vi "FindMovingObjects_Xiang.vi"(6 "Initialize?":bool, 7 "Settings":T2={"Objects"=0, "Threshold"=128, "Reject Border"=FALSE, "Fill Holes"=FALSE, "Min Object Size"=FALSE, "Min Size"=3, "Max Object Size"=FALSE, "Max Size"=100, "Show Search Area"=FALSE, "Show Center"=TRUE, "Show Bounding Box"=TRUE} {"Objects" items=["Bright Objects", "Dark Objects"]; "Threshold" min=1 max=999999999 step=1; "Max Size" min=1 max=999999999 step=1; "Min Size" min=1 max=999999999 step=1}, 8 "Buffer Length":i32=50, 10 "Image Dst":T3, 11 "Image Src":T3) -> (2 "Objects":T1(array[cluster]) {"Aspect Ratio" format="%.2f"; "Orientation" format="%.2f"; "Area" format="%.2f"; "Object Center"."Y" format="%.2f"; "Object Center"."X" format="%.2f"}, 3 "Image Dst Out":T3)   [LabVIEW 2017]
uses:
  <vilib>/vision/Image Controls.llb/IMAQ Image.ctl
  <vilib>/vision/NI_Vision_Development_Module.lvlib
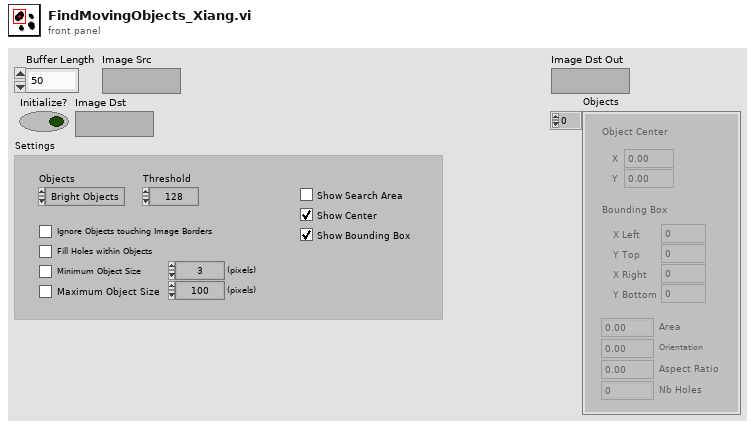
[diagram p1: front panel]
types:
  T1 = cluster{"Object Center":cluster{"X":sgl, "Y":sgl}, "Bounding Box":cluster{"X Left":i32, "Y Top":i32, "X Right":i32, "Y Bottom":i32}, "Area":sgl, "Orientation":sgl, "Aspect Ratio":sgl, "Nb Holes":i32}[]
  T2 = cluster{"Objects":u16, "Threshold":i32, "Reject Border":bool, "Fill Holes":bool, "Min Object Size":bool, "Min Size":i32, "Max Object Size":bool, "Max Size":i32, "Show Search Area":bool, "Show Center":bool, "Show Bounding Box":bool}
  T3 = typedef "IMAQ Image.ctl" = refnum<image>
  T4 = typedef "Image Type" = u32
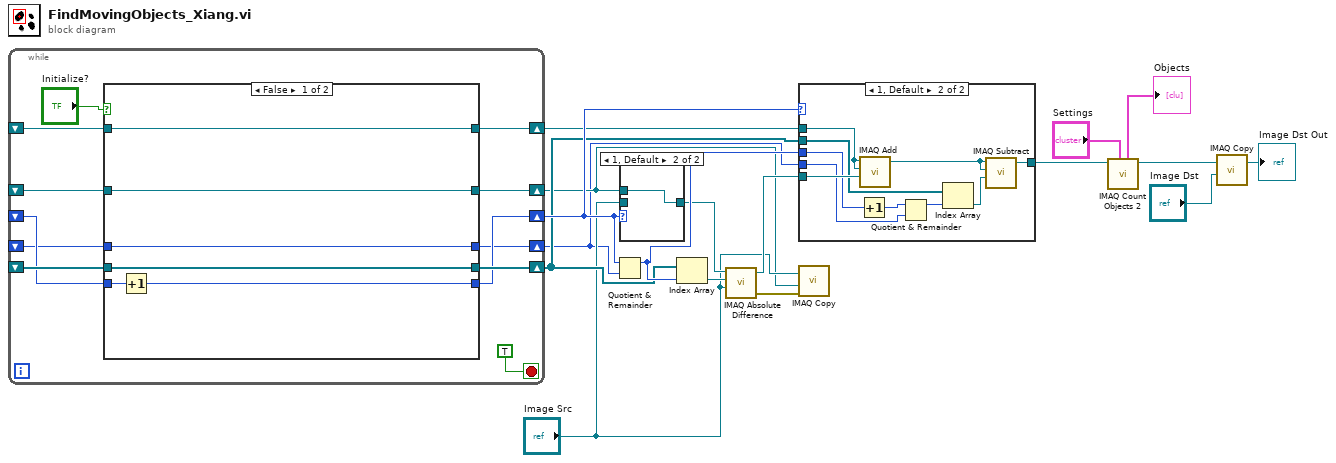
[diagram p0: block diagram]
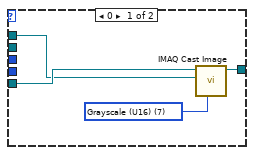
[diagram p2: hidden frame]
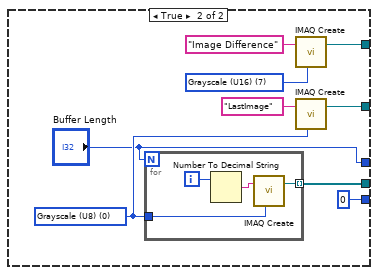
[diagram p4: hidden frame]
diagram:
  n1 = while {
    shift-right: [w28] -> w9
    shift-left: _ -> [w27]
    shift-right: [w25] -> w6
    shift-left: _ -> [w24]
    shift-right: [w23] -> w8
    shift-left: _ -> [w22]
    shift-right: [w20] -> w10
    shift-left: _ -> [w21]
    shift-right: [w19] -> w5
    shift-left: _ -> [w18]
    stop <- TRUE stop-if-true
    n2 = case shown="False" "Initialize?" {
      tunnel: [w35 w44] -> w28
      tunnel: w27 -> [w35 _]
      tunnel: [w34 w42] -> w25
      tunnel: w24 -> [w34 _]
      tunnel: [w33 w38] -> w23
      tunnel: w22 -> [w33 _]
      tunnel: [w31 0] -> w20
      tunnel: w21 -> [w32 _]
      tunnel: [w30 "Buffer Length"] -> w19
      tunnel: w18 -> [w30 _]
      frame False {
        n3 = Increment(x=w32) -> (x+1=w31:i32)
      }
      frame True {
        w41 = T4 7 items=["Grayscale (U8)", "Grayscale (I16)", "Grayscale (SGL)", "Complex (CSG)", "RGB (U32)", "HSL (U32)", "RGB (U64)", "Grayscale (U16)"] ("Image Type")
        w39 = T4 0 items=["Grayscale (U8)", "Grayscale (I16)", "Grayscale (SGL)", "Complex (CSG)", "RGB (U32)", "HSL (U32)", "RGB (U64)", "Grayscale (U16)"] ("Image Type")
        n4 = for {
          N: "Buffer Length" -> [_]
          tunnel: w39 -> [w48]
          tunnel: [w45] -> w44 mode=indexing
          i -> [w47]
          n5 = Number To Decimal String(number=w47) -> (decimal integer string=w46:string)  [unwired: 1 in]
          n6 = call "IMAQ Create"("Image Name"=w46, "Image Type"=w48) -> ("New Image"=w45:T3)  [unwired: 3 in, 1 out]
        }
        n7 = call "IMAQ Create"("Image Name"="Image Difference", "Image Type"=w41) -> ("New Image"=w38:T3)  [unwired: 3 in, 1 out]
        n8 = call "IMAQ Create"("Image Name"="LastImage", "Image Type"=w39) -> ("New Image"=w42:T3)  [unwired: 3 in, 1 out]
      }
    }
  }
  n9 = Quotient & Remainder(x=w10, y=w5) -> (x-y*floor(x/y)=w13:i32)  [unwired: 1 out]
  n10 = case shown="1, Default" w10 {
    tunnel: "Image Src" -> [w49 _]
    tunnel: [w49 w50] -> w12
    tunnel: w6 -> [_ w50]
    frame 0 {
    }
    frame 1, Default {
    }
  }
  n11 = Index Array(array=w9, index=w13) -> (element=w11:T3)
  n12 = call "IMAQ Absolute Difference"("Image Src A"=w12, "Image Dst"=w11, "Image Src B"="Image Src") -> ("Image Dst Out"=w16:T3, "error out"=w17:errorcluster)  [unwired: 4 in]
  n13 = case shown="1, Default" w10 {
    tunnel: w8 -> [w53 w64]
    tunnel: w16 -> [w54 w63]
    tunnel: [w51 w60] -> w15
    tunnel: w9 -> [_ w62]
    tunnel: w13 -> [_ w57]
    tunnel: w5 -> [_ w59]
    frame 0 {
      w52 = T4 7 items=["Grayscale (U8)", "Grayscale (I16)", "Grayscale (SGL)", "Complex (CSG)", "RGB (U32)", "HSL (U32)", "RGB (U64)", "Grayscale (U16)"] ("Image Type")
      n14 = call "IMAQ Cast Image"("Image Type"=w52, "Image Dst"=w53, "Image Src"=w54) -> ("Image Dst Out"=w51:T3)  [unwired: 7 in, 1 out]
    }
    frame 1, Default {
      n15 = Increment(x=w57) -> (x+1=w56:i32)
      n16 = call "IMAQ Add"("Image Src A"=w64, "Image Dst"=w64, "Image Src B"=w63) -> ("Image Dst Out"=w61:T3)  [unwired: 4 in, 1 out]
      n17 = Quotient & Remainder(x=w56, y=w59) -> (x-y*floor(x/y)=w58:i32)  [unwired: 1 out]
      n18 = Index Array(array=w62, index=w58) -> (element=w55:T3)
      n19 = call "IMAQ Subtract"("Image Src A"=w61, "Image Dst"=w61, "Image Src B"=w55) -> ("Image Dst Out"=w60:T3)  [unwired: 4 in, 1 out]
    }
  }
  n20 = call "IMAQ Copy"("error in (no error)"=w17, "Image Dst"=w6, "Image Src"="Image Src") -> ()  [unwired: 3 in, 2 out]
  n21 = call "IMAQ Count Objects 2"("Settings"="Settings", "Image"=w15) -> ("Image Out"=w14:T3, "Objects"=→"Objects":T1)  [unwired: 5 in, 3 out]
  n22 = call "IMAQ Copy"("Image Dst"="Image Dst", "Image Src"=w14) -> ("Image Dst Out"=→"Image Dst Out":T3)  [unwired: 4 in, 1 out]
